vi "bricker_arduino_i2c.vi"(11 "VISA resource name":refnum<visa-resource-name>) -> (1 "VISA resource name out":refnum<visa-resource-name>, 2 "TEMP_DATA":string[](array[string]), 3 "PRESSURE_DATA":string[](array[string]))   [LabVIEW 2022 SP3]
uses:
  <vilib>/regexp/Match Regular Expression.xnode
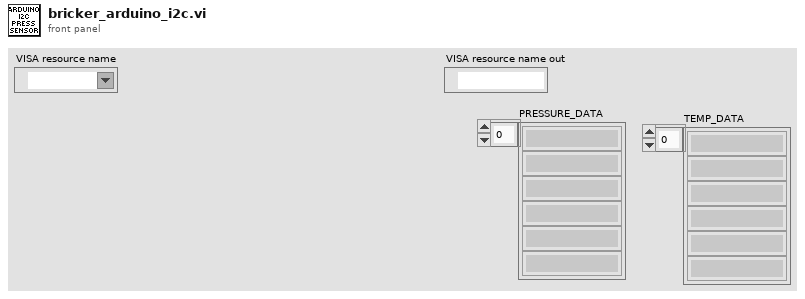
[diagram p1: front panel]
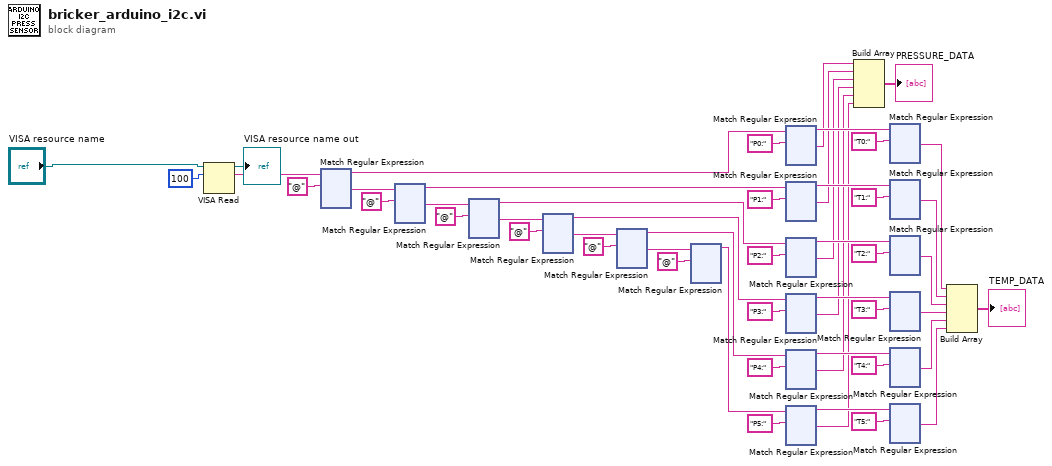
[diagram p0: block diagram]
diagram:
  n1 = VISA Read(VISA resource name="VISA resource name", byte count=u32 100) -> (VISA resource name out=→"VISA resource name out":refnum<visa-resource-name>, read buffer=w52:string)  [unwired: 1 in, 2 out]
  n2 = xnode "Match Regular Expression"("input string"=w52, "regular expression"="@") -> ("before match"=w49:string, "after match"=w31:string)  [unwired: 4 in, 3 out]
  n3 = xnode "Match Regular Expression"("input string"=w31, "regular expression"="@") -> ("before match"=w44:string, "after match"=w30:string)  [unwired: 4 in, 3 out]
  n4 = xnode "Match Regular Expression"("input string"=w30, "regular expression"="@") -> ("before match"=w39:string, "after match"=w29:string)  [unwired: 4 in, 3 out]
  n5 = xnode "Match Regular Expression"("input string"=w29, "regular expression"="@") -> ("before match"=w34:string, "after match"=w18:string)  [unwired: 4 in, 3 out]
  n6 = xnode "Match Regular Expression"("input string"=w18, "regular expression"="@") -> ("before match"=w26:string, "after match"=w17:string)  [unwired: 4 in, 3 out]
  n7 = xnode "Match Regular Expression"("input string"=w17, "regular expression"="@") -> ("before match"=w21:string)  [unwired: 4 in, 4 out]
  n8 = xnode "Match Regular Expression"("input string"=w49, "regular expression"="P0:") -> ("before match"=w47:string, "after match"=w9:string)  [unwired: 4 in, 3 out]
  n9 = xnode "Match Regular Expression"("input string"=w44, "regular expression"="P1:") -> ("before match"=w46:string, "after match"=w8:string)  [unwired: 4 in, 3 out]
  n10 = xnode "Match Regular Expression"("input string"=w39, "regular expression"="P2:") -> ("before match"=w37:string, "after match"=w7:string)  [unwired: 4 in, 3 out]
  n11 = xnode "Match Regular Expression"("input string"=w34, "regular expression"="P3:") -> ("before match"=w36:string, "after match"=w6:string)  [unwired: 4 in, 3 out]
  n12 = xnode "Match Regular Expression"("input string"=w26, "regular expression"="P4:") -> ("before match"=w24:string, "after match"=w5:string)  [unwired: 4 in, 3 out]
  n13 = xnode "Match Regular Expression"("input string"=w21, "regular expression"="P5:") -> ("before match"=w23:string, "after match"=w4:string)  [unwired: 4 in, 3 out]
  n14 = Build Array(w9, w8, w7, w6, w5, w4) -> (→"PRESSURE_DATA":string[])
  n15 = xnode "Match Regular Expression"("input string"=w47, "regular expression"="T0:") -> ("after match"=w16:string)  [unwired: 4 in, 4 out]
  n16 = xnode "Match Regular Expression"("input string"=w46, "regular expression"="T1:") -> ("after match"=w15:string)  [unwired: 4 in, 4 out]
  n17 = xnode "Match Regular Expression"("input string"=w37, "regular expression"="T2:") -> ("after match"=w14:string)  [unwired: 4 in, 4 out]
  n18 = xnode "Match Regular Expression"("input string"=w36, "regular expression"="T3:") -> ("after match"=w13:string)  [unwired: 4 in, 4 out]
  n19 = xnode "Match Regular Expression"("input string"=w24, "regular expression"="T4:") -> ("after match"=w12:string)  [unwired: 4 in, 4 out]
  n20 = xnode "Match Regular Expression"("input string"=w23, "regular expression"="T5:") -> ("after match"=w11:string)  [unwired: 4 in, 4 out]
  n21 = Build Array(w16, w15, w14, w13, w12, w11) -> (→"TEMP_DATA":string[])
